vi "set_output_on.vi"(8 "error in":errorcluster, 11 "VISA resource name":refnum<visa-resource-name>="COM1") -> (0 "error out":errorcluster, 3 "Response":string)   [LabVIEW 2020]
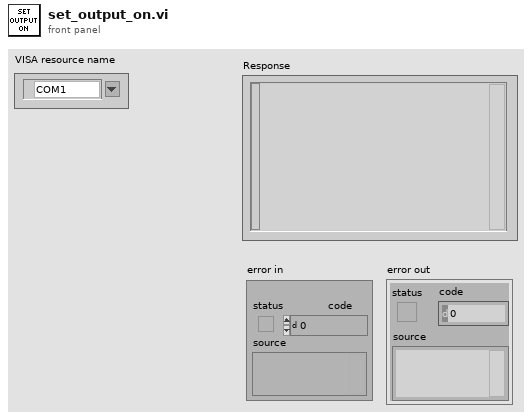
[diagram p1: front panel]
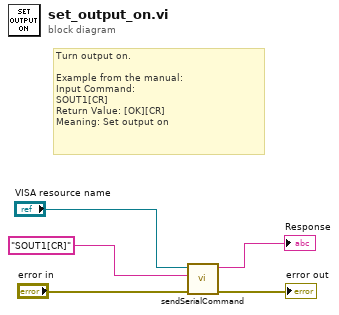
[diagram p0: block diagram]
diagram:
  # "Turn output on.\n\nExample from the manual:\nInput Command:\nSOUT1[CR]\nReturn Value: [OK][CR]\nMeaning: Set output on"
  n1 = call "sendSerialCommand.vi"("error in (no error)"="error in", "Command"="SOUT1[CR]", "VISA resource name"="VISA resource name") -> ("error out"=→"error out":errorcluster, "Response"=→"Response":string)  [unwired: 7 in]
